vi "power value to sting.vi"(9 "Power":T1) -> (10 "power string":string)   [LabVIEW 2011]
uses:
  Power_config.ctl
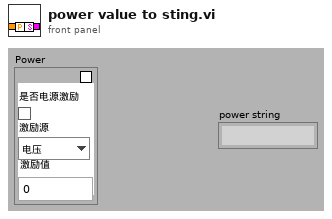
[diagram p1: front panel]
types:
  T1 = typedef "Power_config.ctl" = cluster{"power_en":bool, "Mode":enum16{"电压", "电流"}, "value":dbl, "Boolean":bool}
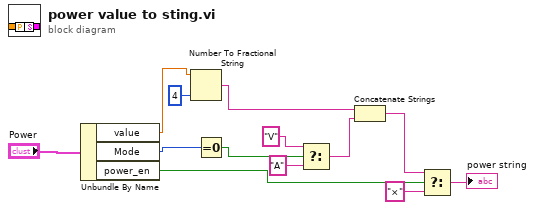
[diagram p0: block diagram]
diagram:
  n1 = Unbundle By Name("Power") -> ("value"=w11:dbl, "Mode"=w12:enum16{"电压", "电流"}, "power_en"=w6:bool)
  n2 = Number To Fractional String(number=w11, precision (6)=i16 4) -> (F-format string=w5:string)  [unwired: 2 out]
  n3 = Equal To 0?(x=w12) -> (x = 0?=w9:bool)
  n4 = Select(t="V", s=w9, f="A") -> (s? t:f=w4:string)
  n5 = Concatenate Strings(w5, w4) -> (w3:string)
  n6 = Select(t=w3, s=w6, f="×") -> (s? t:f=→"power string":string)
